vi "BRig_dataLC_Loop1_c.vi"() -> (2 "output_Loop1_c":i32)   [LabVIEW 2014]
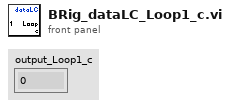
[diagram p1: front panel]
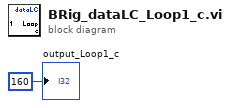
[diagram p0: block diagram]
diagram:
  "output_Loop1_c" <- 160 ("output_iBlock")
